vi "createControl.vi"(8 "error in (no error)":errorcluster, 10 "LibraryInfo":T1, 11 "Topic in":refnum<class "Topic.lvclass">) -> (0 "error out":errorcluster, 3 "Topic out":refnum<class "Topic.lvclass">)   [LabVIEW 2012, in "Topic.lvclass"]
uses:
  Topic.lvclass
  Typedefs/LibraryInfo.ctl
  Topic.lvclass/Topic.ctl
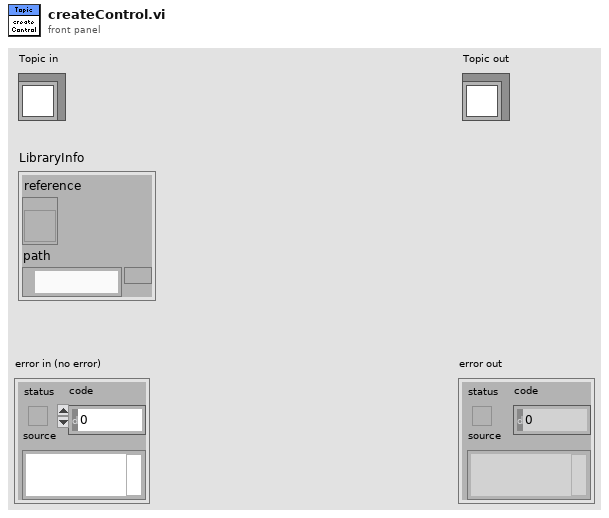
[diagram p1: front panel]
types:
  T1 = typedef "LibraryInfo.ctl" = cluster{"reference":refnum<vi>, "path":path}
  T2 = enum32{"not a control VI", "control", "typedef", "strict typedef"}
  T3 = enum32{"invalid VI type", "Standard VI", "Control VI", "Global VI", "Polymorphic VI", "Configuration VI", "SubSystem", "Facade VI", "Method VI", "Statechart Diagram VI"}
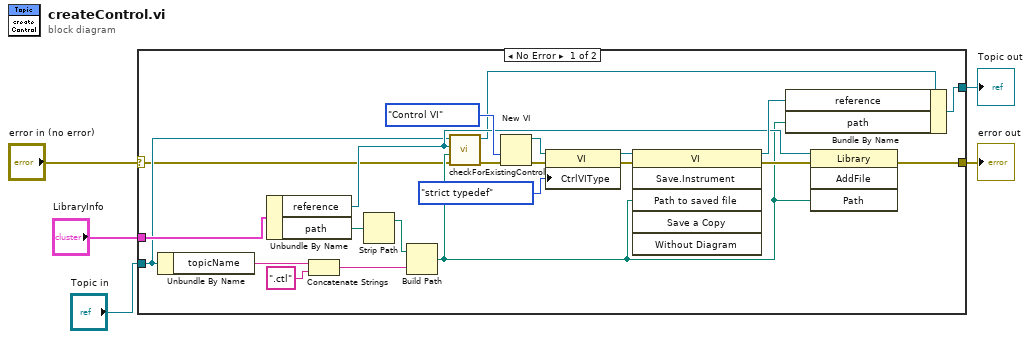
[diagram p0: block diagram]
diagram:
  n1 = case shown="No Error" "error in (no error)" {
    selector: "error in (no error)" -> [w7 w29]
    tunnel: [w14 w29] -> w4
    tunnel: [w17 w28] -> w2
    tunnel: "Topic in" -> [w9 w28]
    tunnel: "LibraryInfo" -> [w22 _]
    frame No Error {
      n2 = Unbundle By Name(w9) -> ("topicName"=w21:string)
      n3 = Unbundle By Name(w22) -> ("reference"=w11:refnum<vi>, "path"=w19:path)
      n4 = Concatenate Strings(w21, ".ctl" ("string")) -> (w25:string)
      n5 = Strip Path(path=w19) -> (stripped path=w20:path)  [unwired: 1 out]
      n6 = Build Path(base path=w20, name or relative path=w25) -> (appended path=w10:path)
      n7 = call "checkForExistingControl.vi"("error in (no error)"=w7, "controlPath"=w10, "libraryRef"=w11, "Topic in"=w9) -> ("error out"=w6:errorcluster, "Topic out"=w8:refnum<class "Topic.lvclass">)  [unwired: 6 in]
      n8 = New VI(8:w6, 9:T3."Control VI" ("vi type (standard vi)")) -> (0:w15:errorcluster, 3:w24:refnum<vi>)  [unwired: 5 in]
      n9 = property class="VI"(reference=w24, error in=w15, "CtrlVIType"=T2."strict typedef" ("Control VI Type")) -> (reference out=w12:refnum<vi>, error out=w13:errorcluster)
      n10 = invoke class="VI" method="Save.Instrument"(reference=w12, error in=w13, "Path to saved file"=w10) -> (reference out=w18:refnum<vi>, error out=w16:errorcluster)  [unwired: 3 in, 4 out]
      n11 = Bundle By Name(cluster=w8, "reference"=w18, "path"=w10) -> (w17:refnum<class "Topic.lvclass">)
      n12 = invoke class="Library" method="AddFile"(reference=w11, error in=w16, "Path"=w10) -> (error out=w14:errorcluster)  [unwired: 1 in, 3 out]
    }
    frame Error {
    }
  }
  "error out" <- w4
  "Topic out" <- w2
